vi "RIOPhysicalNameToCardChannelNumbers.vi"(3 "Channel Name":string) -> (0 "Channel #":string, 1 "Card #":string)   [LabVIEW 2015]
doc: "Takes the RIO [card.channel] physical name (comes in as a string), and outputs the card/channel # as a string. Used for looped tagging."
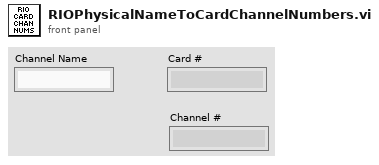
[diagram p1: front panel]
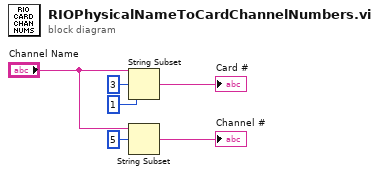
[diagram p0: block diagram]
diagram:
  n1 = String Subset(string="Channel Name", offset (0)=3, length (rest)=1 ("length (rest)")) -> (substring=→"Card #":string)
  n2 = String Subset(string="Channel Name", offset (0)=5) -> (substring=→"Channel #":string)  [unwired: 1 in]
